vi "visualyze_audio_data.vi"(8 "error in (no error)":errorcluster, 10 "audio data":waveform(dbl)[](array[waveform]), 11 "Button refs In":T1) -> (0 "error out":errorcluster)   [LabVIEW 2021]
uses:
  CTLs/ButtonRefs.ctl
  CTLs/playback status.ctl
  FGVs/FGVstates.ctl
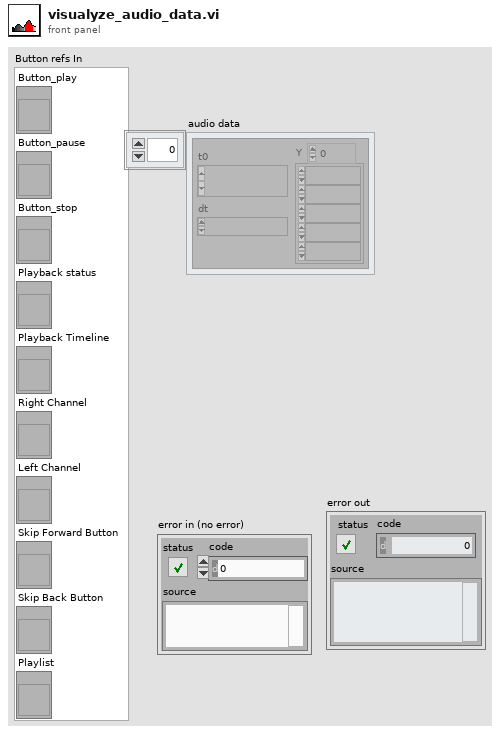
[diagram p1: front panel]
types:
  T1 = typedef "ButtonRefs.ctl" = cluster{"Button_play":refnum<vi>, "Button_pause":refnum<vi>, "Button_stop":refnum<vi>, "Playback status":refnum<vi>, "Playback Timeline":refnum<vi>, "Right Channel":refnum<vi>, "Left Channel":refnum<vi>, "Skip Forward Button":refnum<vi>, "Skip Back Button":refnum<vi>, "Playlist":refnum<vi>}
  T2 = typedef "FGVstates.ctl" = enum16{"Init", "Set", "Get", "De-Init"}
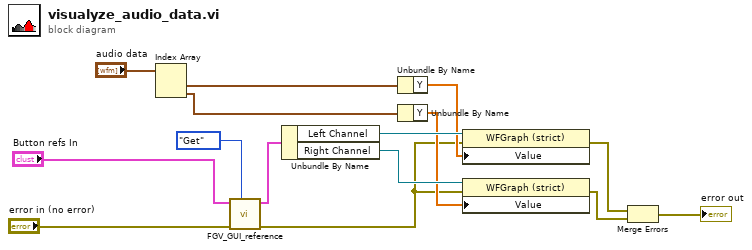
[diagram p0: block diagram]
diagram:
  n1 = Index Array(array="audio data") -> (element #1=w9:waveform(dbl), element #2=w6:waveform(dbl))  [unwired: 2 in]
  n2 = call "FGV_GUI_reference.vi"("FGV states"=FGVstates."Get", "error in (no error)"="error in (no error)", "Button refs In"="Button refs In") -> ("error out"=w5:errorcluster, "Button refs Out"=w13:T1)  [unwired: 7 in]
  n3 = Unbundle By Name(w13) -> ("Left Channel"=w12:refnum<vi>, "Right Channel"=w11:refnum<vi>)
  n4 = Unbundle By Name(w9) -> ("Y"=w8:dbl[])
  n5 = Unbundle By Name(w6) -> ("Y"=w7:dbl[])
  n6 = property class="WFGraph (strict)"(reference=w12, error in=w5, "Value"=w8) -> (error out=w4:errorcluster)  [unwired: 1 out]
  n7 = property class="WFGraph (strict)"(reference=w11, error in=w5, "Value"=w7) -> (error out=w2:errorcluster)  [unwired: 1 out]
  n8 = Merge Errors(w4, w2) -> (→"error out":errorcluster)
